vi "Attenuator Execute Test.vi"(4 "PFLabel":refnum<vi>, 6 "Driver Refs":T1, 8 "error in (no error)":errorcluster, 9 "Test Parameters In":T6={"Stimulus"={"ATT Stimulus"={"Normalize"=TRUE, "Value (dB)"=0.0}, "VNA Stimulus"={"Use Instrument Settings"=FALSE, "Blank Frequencies"=FALSE, "Sweep Type"=enum."Linear", "Sweep"={"Fstart"=500.0, "Fstop"=1500.0, "Units"=enum."MHz", "Points"=201}, "Power (dBm)"=999.0, "IFBW (Hz)"=-1.0, "Sweep Time (s)"=-1.0, "Calibration"={"State"=FALSE, "String"=""}}}, "Measurement"={"Step (dB)"=enum."0.25", "Start (dB)"=0.0, "Stop (dB)"=31.75}, "Limit"={"Maximum Error"=0.3}, "Normalization"={"Normalized?"=FALSE, "Normalization Values (dB)"=[]}} {"Stimulus"."VNA Stimulus"."Sweep Time (s)" format="%.3g"}, 11 "Empty Measurement Values":T5) -> (0 "error out":errorcluster, 1 "Test Parameters Out":T6={"Stimulus"={"ATT Stimulus"={"Normalize"=TRUE, "Value (dB)"=0.0}, "VNA Stimulus"={"Use Instrument Settings"=FALSE, "Blank Frequencies"=FALSE, "Sweep Type"=enum."Linear", "Sweep"={"Fstart"=500.0, "Fstop"=1500.0, "Units"=enum."MHz", "Points"=201}, "Power (dBm)"=999.0, "IFBW (Hz)"=-1.0, "Sweep Time (s)"=-1.0, "Calibration"={"State"=FALSE, "String"=""}}}, "Measurement"={"Step (dB)"=enum."0.25", "Start (dB)"=0.0, "Stop (dB)"=31.75}, "Limit"={"Maximum Error"=0.3}, "Normalization"={"Normalized?"=FALSE, "Normalization Values (dB)"=[]}} {"Stimulus"."VNA Stimulus"."Sweep Time (s)" format="%.3g"}, 2 "Passed?":bool, 3 "Measurement Values":T5, 5 "Done?":bool)   [LabVIEW 2011]
uses:
  TypeDefs/Attenuator Test Parameters.ctl
  TypeDefs/Attenuator Stimulus Parameters.ctl
  TypeDefs/Attenuator ATT Stimulus.ctl
  TypeDefs/Attenuator VNA Stimulus.ctl
  S Parameter/TypeDefs/SP Frequency Units.ctl
  TypeDefs/Attenuator VNA Calibration State.ctl
  TypeDefs/Attenuator Measurement Cluster.ctl
  TypeDefs/Attenuator Limit.ctl
  TypeDefs/Attenuator Calibration State.ctl
  TypeDefs/Attenuator Driver Refs.ctl
  drivers/ATT/ATT Driver Ref.ctl
  drivers/VNA/VNA Driver Ref.ctl
  drivers/SNA/SNA Driver Ref.ctl
  TypeDefs/Attenuator Measurement Values.ctl
  TypeDefs/Attenuator Parameter to Measure.ctl
  S Parameter/TypeDefs/SP Parameter.ctl
  S Parameter/TypeDefs/SP Measurement Format.ctl
  drivers/VNA/VNA Command.ctl
  drivers/ATT/ATT Command.ctl
panel:
  out "Driver Refs":T1
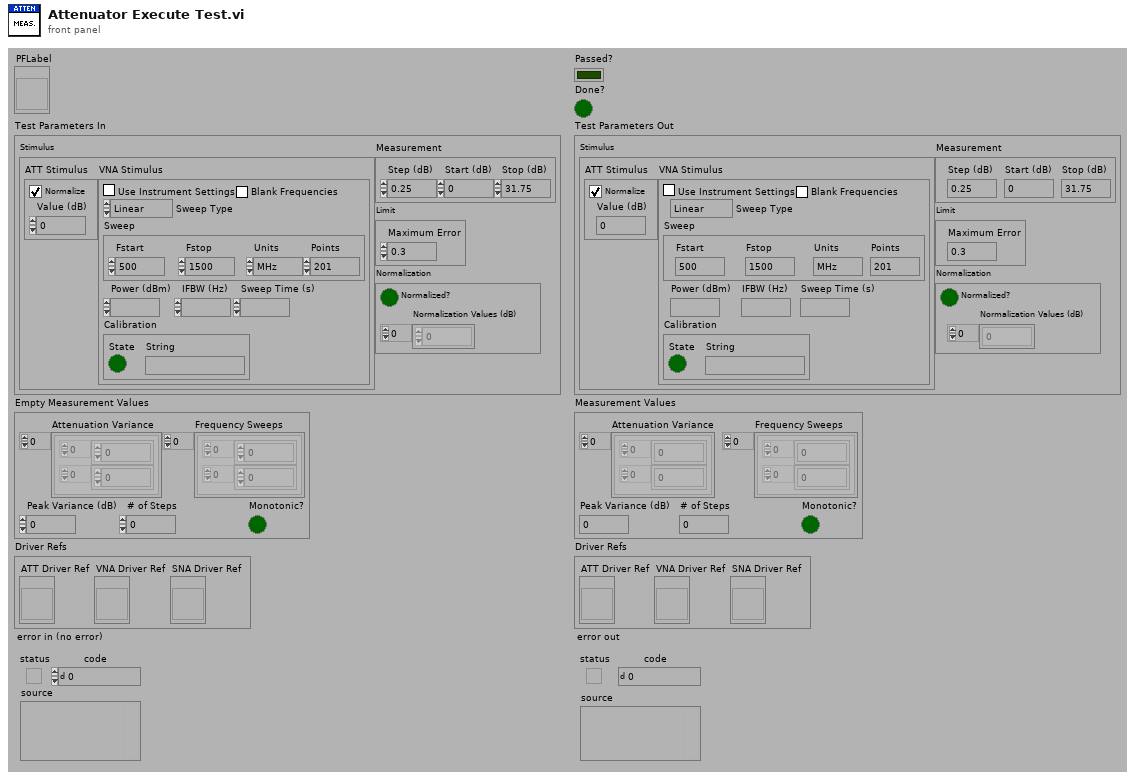
[diagram p1: front panel]
types:
  T1 = typedef "Attenuator Driver Refs.ctl" = cluster{"ATT Driver Ref":T2, "VNA Driver Ref":T3, "SNA Driver Ref":T4}
  T2 = typedef "ATT Driver Ref.ctl" = refnum<vi>
  T3 = typedef "VNA Driver Ref.ctl" = refnum<vi>
  T4 = typedef "SNA Driver Ref.ctl" = refnum<vi>
  T5 = typedef "Attenuator Measurement Values.ctl" = cluster{"# of Steps":i32, "Attenuation Variance":cluster{"X":dbl[], "Y":dbl[]}[], "Frequency Sweeps":cluster{"X":dbl[], "Y":dbl[]}[], "Peak Variance (dB)":dbl, "Monotonic?":bool}
  T6 = typedef "Attenuator Test Parameters.ctl" = cluster{"Stimulus":T7, "Measurement":T12, "Limit":T13, "Normalization":T14}
  T7 = typedef "Attenuator Stimulus Parameters.ctl" = cluster{"ATT Stimulus":T8, "VNA Stimulus":T9}
  T8 = typedef "Attenuator ATT Stimulus.ctl" = cluster{"Normalize":bool, "Value (dB)":dbl}
  T9 = typedef "Attenuator VNA Stimulus.ctl" = cluster{"Use Instrument Settings":bool, "Blank Frequencies":bool, "Sweep Type":enum32{"Linear", "Logarithmic", "List", "Power", "CW"}, "Sweep":cluster{"Fstart":dbl, "Fstop":dbl, "Units":T10, "Points":i32}, "Power (dBm)":dbl, "IFBW (Hz)":dbl, "Sweep Time (s)":dbl, "Calibration":T11}
  T10 = typedef "SP Frequency Units.ctl" = enum16{"Hz", "kHz", "MHz", "GHz", "Points"}
  T11 = typedef "Attenuator VNA Calibration State.ctl" = cluster{"State":bool, "String":string}
  T12 = typedef "Attenuator Measurement Cluster.ctl" = cluster{"Step (dB)":enum16{"0.25", "0.50", "1.00"}, "Start (dB)":dbl, "Stop (dB)":dbl}
  T13 = typedef "Attenuator Limit.ctl" = cluster{"Maximum Error":dbl}
  T14 = typedef "Attenuator Calibration State.ctl" = cluster{"Normalized?":bool, "Normalization Values (dB)":dbl[]}
  T15 = typedef "ATT Command.ctl" = enum16{"LOAD", "INITIALIZE", "PRESET", "SET STIMULUS", "GET STIMULUS", "GET CALIBRATION", "CALIBRATE", "GET INFO", "RELEASE", "UNLOAD"}
  T16 = typedef "VNA Command.ctl" = enum16{"LOAD", "INITIALIZE", "PRESET", "GET STIMULUS", "SET STIMULUS", "GET CALIBRATION", "CALIBRATE", "RESTORE", "MEASURE", "RELEASE", "UNLOAD", "CONFIRM", "SORT"}
  T17 = typedef "Attenuator Parameter to Measure.ctl" = cluster{"Channel":i8, "Parameter":T18, "Calibration":T11, "Display Format":T19, "Pass?":bool}
  T18 = typedef "SP Parameter.ctl" = cluster{"Stimulus Port":i8, "Response Port":i8}
  T19 = typedef "SP Measurement Format.ctl" = enum32{"Log Mag", "Phase", "Delay", "Smith (R+jX)", "Polar (Re/Im)", "Linear Mag", "SWR", "Real", "Imaginary", "Smith (Lin/Phase)", "Smith (Log/Phase)", "Smith (Real/Imag)", "Smith (G+jB)", "Polar (Lin/Phase)", "Polar (Log/Phase)", "Expanded Phase", "Positive Phase", "Inverted Smith", "Unwrapped Phase", "Power Out", "Power In", "Linear Mag/Phase", "Log Mag/Phase", "Real/Imaginary"}
  T20 = typedef "SP Data.ctl" = cluster{"F0":dbl, "dF":dbl, "Data":cdb[][]}
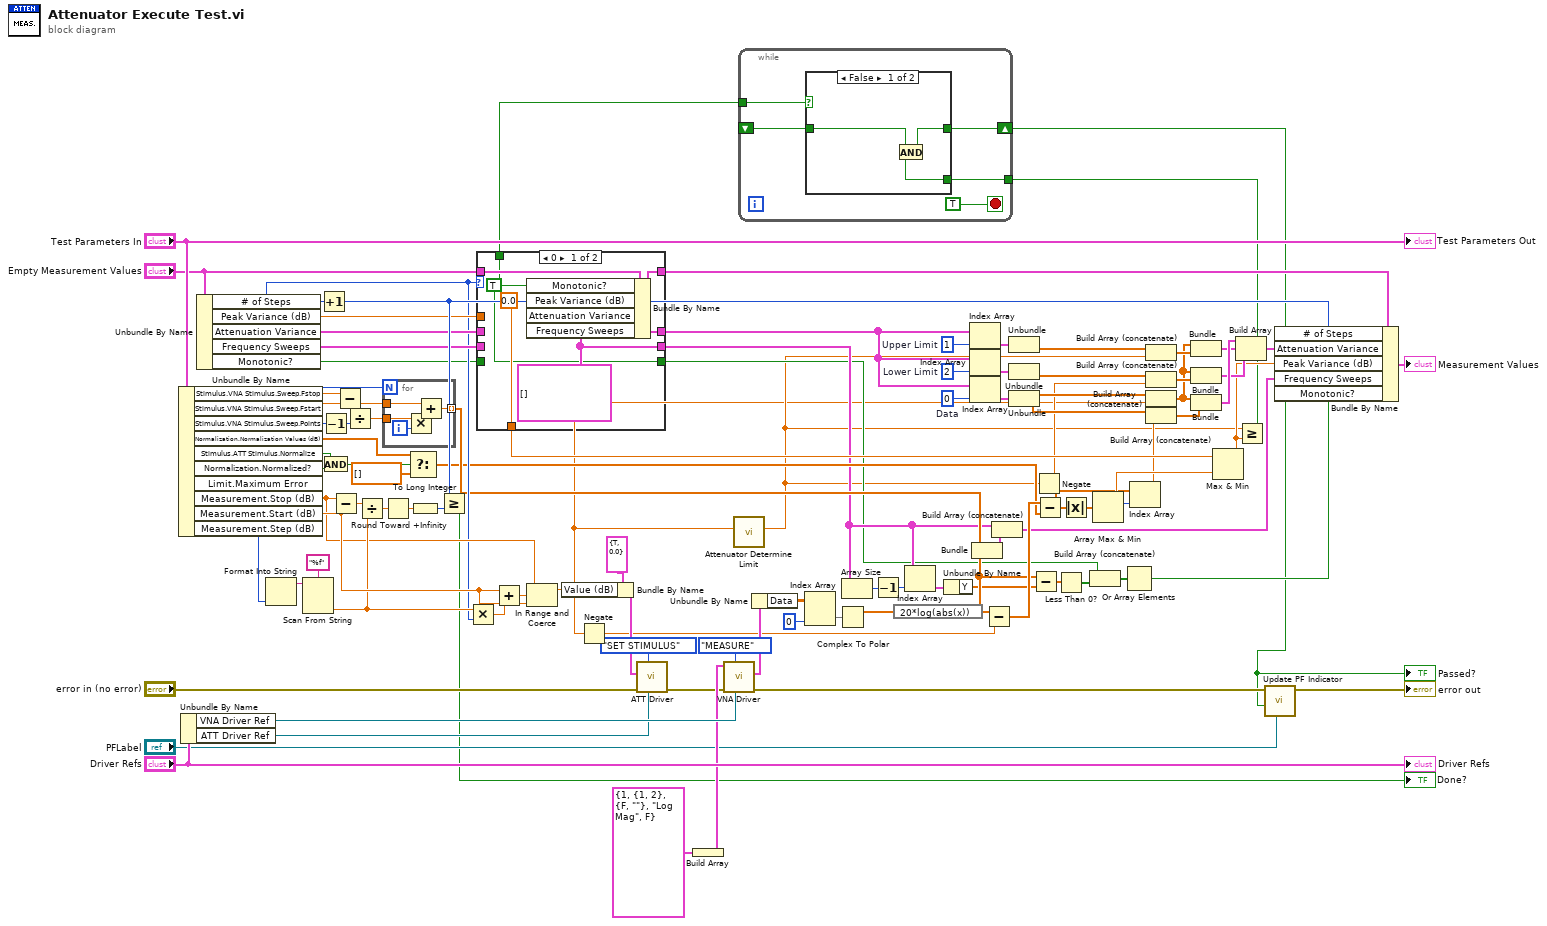
[diagram p0: block diagram]
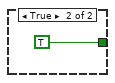
[diagram p2: hidden frame]
diagram:
  w50 = 1  # Upper Limit
  w57 = 0  # Data
  w58 = 2  # Lower Limit
  n1 = Unbundle By Name("Test Parameters In") -> ("Stimulus.VNA Stimulus.Sweep.Fstop"=w35:dbl, "Stimulus.VNA Stimulus.Sweep.Fstart"=w29:dbl, "Stimulus.VNA Stimulus.Sweep.Points"=w26:i32, "Normalization.Normalization Values (dB)"=w87:dbl[], "Stimulus.ATT Stimulus.Normalize"=w36:bool, "Normalization.Normalized?"=w89:bool, "Measurement.Stop (dB)"=w93:dbl, "Measurement.Start (dB)"=w96:dbl, "Measurement.Step (dB)"=w82:enum16{"0.25", "0.50", "1.00"})  [unwired: 1 out]
  n2 = Unbundle By Name("Driver Refs") -> ("VNA Driver Ref"=w102:T3, "ATT Driver Ref"=w101:T2)
  n3 = Unbundle By Name("Empty Measurement Values") -> ("# of Steps"=w37:i32, "Peak Variance (dB)"=w72:dbl, "Attenuation Variance"=w71:cluster{"X":dbl[], "Y":dbl[]}[], "Frequency Sweeps"=w38:cluster{"X":dbl[], "Y":dbl[]}[], "Monotonic?"=w16:bool)
  n4 = Format Into String(w82) -> (resulting string=w81:string)  [unwired: 3 in, 1 out]
  n5 = Scan From String(format string="%f", input string=w81) -> (output 1=w94:dbl)  [unwired: 3 in, 3 out]
  n6 = Increment(x=w37) -> (x+1=w76:i32)
  n7 = Decrement(x=w26) -> (x-1=w27:i32)
  n8 = And(x=w36, y=w89) -> (x .and. y?=w88:bool)
  n9 = Subtract(x=w93, y=w96) -> (x-y=w99:dbl)
  n10 = Subtract(x=w35, y=w29) -> (x-y=w34:dbl)
  n11 = Divide(x=w34, y=w27) -> (x/y=w33:dbl)
  n12 = Divide(x=w99, y=w94) -> (x/y=w98:dbl)
  n13 = for {
    N: w26 -> [_]
    tunnel: w29 -> [w104]
    tunnel: w33 -> [w107]
    tunnel: [w103] -> w32 mode=indexing
    i -> [w106]
    n14 = Multiply(x=w107, y=w106) -> (x*y=w105:dbl)
    n15 = Add(x=w104, y=w105) -> (x+y=w103:dbl)
  }
  n16 = Round Toward +Infinity(x=w98) -> (ceil(x): smallest int >= x=w77:dbl)
  n17 = Select(t=w87, s=w88, f=dbl[] []) -> (s? t:f=w25:dbl[])
  n18 = To Long Integer(number=w77) -> (32bit integer=w75:i32)
  n19 = Greater Or Equal?(x=w76, y=w75) -> (x >= y?=→"Done?":bool)
  n20 = Multiply(x=w94, y=w37) -> (x*y=w67:dbl)
  n21 = case shown="0" w37 {
    tunnel: [w109 w115] -> w80
    tunnel: "Empty Measurement Values" -> [w112 w117]
    tunnel: [w111 w117] -> w78
    tunnel: [w110 w116] -> w73
    tunnel: w72 -> [_ w116]
    tunnel: w71 -> [_ w115]
    tunnel: w38 -> [_ w114]
    tunnel: [w109 w114] -> w19
    tunnel: w16 -> [_ w113]
    tunnel: [w108 w113] -> w12
    tunnel: [w108 _] -> w3
    frame 0 {
      w108 = TRUE ("Monotonic?")
      w110 = 0.0 ("Peak Variance (dB)")
      w109 = cluster{dbl[], dbl[]}[] [] ("Value")
      n22 = Bundle By Name(cluster=w112, "Monotonic?"=w108, "Peak Variance (dB)"=w110, "Attenuation Variance"=w109, "Frequency Sweeps"=w109) -> (w111:T5)
    }
    frame Default {
    }
  }
  n23 = Add(x=w96, y=w67) -> (x+y=w66:dbl)
  n24 = In Range and Coerce(upper limit=w93, x=w66, lower limit=w96) -> (coerced(x)=w4:dbl)  [unwired: 1 out]
  n25 = Bundle By Name(cluster=T8 {"Normalize"=TRUE, "Value (dB)"=0.0} ("ATT Value In"), "Value (dB)"=w4) -> (w64:T8)
  n26 = Negate(x=w4) -> (-x=w11:dbl)
  n27 = call "ATT Driver.vi"("Drv Refnum"=w101, "ATT Command"=ATT_Command."SET STIMULUS" ("DMM Command"), "error in (no error)"="error in (no error)", "ATT Value In"=w64) -> ("error out"=w68:errorcluster)  [unwired: 4 in, 3 out]
  n28 = Build Array(T17 {"Channel"=1, "Parameter"={"Stimulus Port"=1, "Response Port"=2}, "Calibration"={"State"=FALSE, "String"=""}, "Display Format"=enum."Log Mag", "Pass?"=FALSE} ("Parameter to Measure")) -> (w91:T17[])
  n29 = call "VNA Driver.vi"("Drv Refnum"=w102, "VNA Command"=VNA_Command."MEASURE", "error in (no error)"=w68, "Parameters to Measure"=w91) -> ("error out"=w40:errorcluster, "SP Data"=w59:T20)  [unwired: 3 in, 3 out]
  n30 = call "Attenuator Determine Limit.vi"("Attenuation Value (0 dB)"=w4) -> ("Maximum Error (dB)"=w5:dbl)  [unwired: 10 in]
  n31 = Unbundle By Name(w59) -> ("Data"=w61:cdb[][])
  n32 = Index Array(array=w61, index (col)=0 ("disabled index (col)")) -> (element=w63:cdb[])  [unwired: 1 in]
  n33 = Complex To Polar(r * e^(i*theta)=w63) -> (r=w60:dbl[])  [unwired: 1 out]
  n34 = Array Size(array=w19) -> (size(s)=w20:i32)
  n35 = Decrement(x=w20) -> (x-1=w7:i32)
  n36 = expression code="20*log(abs(x))"(w60) -> (w21:dbl[])
  n37 = Index Array(array=w19, index=w7) -> (element=w18:cluster{"X":dbl[], "Y":dbl[]})
  n38 = Unbundle By Name(w18) -> ("Y"=w17:dbl[])
  n39 = Index Array(array=w80, index=w50) -> (element=w56:cluster{"X":dbl[], "Y":dbl[]})
  n40 = Index Array(array=w80, index=w58) -> (element=w53:cluster{"X":dbl[], "Y":dbl[]})
  n41 = Index Array(array=w80, index=w57) -> (element=w54:cluster{"X":dbl[], "Y":dbl[]})
  n42 = Bundle(w32, w21) -> (w31:cluster{dbl[], dbl[]})  [unwired: 1 in]
  n43 = Subtract(x=w21, y=w11) -> (x-y=w39:dbl[])
  n44 = Build Array (concatenate)(w19, w31) -> (w30:cluster{"X":dbl[], "Y":dbl[]}[])
  n45 = Unbundle(w56) -> ("Y"=w51:dbl[])  [unwired: 1 out]
  n46 = Unbundle(w53) -> ("Y"=w52:dbl[])  [unwired: 1 out]
  n47 = Unbundle(w54) -> ("X"=w55:dbl[], "Y"=w49:dbl[])
  n48 = Subtract(x=w21, y=w17) -> (x-y=w22:dbl[])
  n49 = Negate(x=w5) -> (-x=w48:dbl)
  n50 = Subtract(x=w39, y=w25) -> (x-y=w10:dbl[])
  n51 = Less Than 0?(x=w22) -> (x < 0?=w15:bool[])
  n52 = Absolute Value(x=w10) -> (abs(x)=w24:dbl[])
  n53 = Build Array (concatenate)(w12, w15) -> (w14:bool[])
  n54 = Array Max & Min(array=w24) -> (max value=w23:dbl, max index (indices)=w9:i32)  [unwired: 2 out]
  n55 = Or Array Elements(Boolean array=w14) -> (logical OR=w13:bool)
  n56 = Index Array(array=w10, index=w9) -> (element=w8:dbl)
  n57 = Build Array (concatenate)(w51, w5) -> (w46:dbl[])
  n58 = Build Array (concatenate)(w52, w48) -> (w45:dbl[])
  n59 = Build Array (concatenate)(w55, w4) -> (w44:dbl[])
  n60 = Build Array (concatenate)(w49, w8) -> (w47:dbl[])
  n61 = Bundle(w44, w46) -> (w42:cluster{dbl[], dbl[]})  [unwired: 1 in]
  n62 = Bundle(w44, w45) -> (w41:cluster{dbl[], dbl[]})  [unwired: 1 in]
  n63 = Bundle(w44, w47) -> (w43:cluster{dbl[], dbl[]})  [unwired: 1 in]
  n64 = Max & Min(x=w73, y=w23) -> (max(x,y)=w6:dbl)  [unwired: 1 out]
  n65 = Build Array(w43, w42, w41) -> (w84:cluster{dbl[], dbl[]}[])
  n66 = Greater Or Equal?(x=w5, y=w6) -> (x >= y?=w2:bool)
  n67 = while {
    shift-right: [w121] -> w1
    shift-left: _ -> [w122]
    tunnel: w3 -> [w120]
    tunnel: w2 -> [w118]
    stop <- TRUE stop-if-true
    n68 = case shown="False" w120 {
      tunnel: w122 -> [w125 _]
      tunnel: [w123 TRUE] -> w121
      tunnel: w118 -> [w124 _]
      frame False {
        n69 = And(x=w125, y=w124) -> (x .and. y?=w123:bool)
      }
      frame True {
      }
    }
  }
  "Passed?" <- w1
  n70 = call "Update PF Indicator.vi"("PFLabel"="PFLabel", "Pass? (f)"=w1, "error in (no error)"=w40) -> ("error out"=→"error out":errorcluster)  [unwired: 1 in, 7 out]
  n71 = Bundle By Name(cluster=w78, "# of Steps"=w76, "Attenuation Variance"=w84, "Peak Variance (dB)"=w6, "Frequency Sweeps"=w30, "Monotonic?"=w13) -> (→"Measurement Values":T5)
  "Test Parameters Out" <- "Test Parameters In"
  "Driver Refs" <- "Driver Refs"
